vi "ziSetValueDouble.vi"(3 "Error In":errorcluster, 4 "Value":dbl, 5 "Path":string, 6 "Handle In":T1 {"Handle" format="0x%08x"; "Conn" format="0x%08x"}) -> (0 "Error Out":errorcluster, 2 "Handle Out":T1 {"Handle" format="0x%08x"; "Conn" format="0x%08x"})   [LabVIEW 2018, in "Zurich Instruments LabOne.lvlib"]
doc: "This vi sets values to the nodes specified in Path to Value. More than one node can be set if a wildcard is used in Path."
uses:
  Zurich Instruments LabOne.lvlib
  ziTypeHandle.ctl
  ziLV32.dll
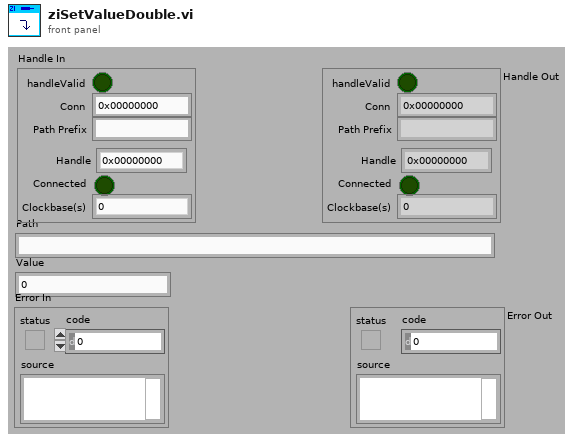
[diagram p1: front panel]
types:
  T1 = typedef "Zurich Instruments LabOne.lvlib/ziTypeHandle.ctl" = cluster{"handleValid":bool, "Conn":u64, "Path Prefix":string, "Handle":u64, "Connected":bool, "Clockbase(s)":dbl}
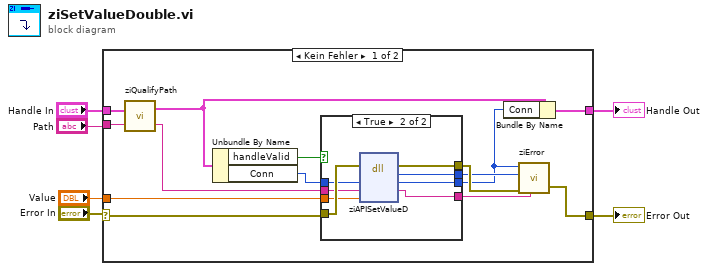
[diagram p0: block diagram]
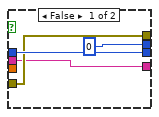
[diagram p2: hidden frame]
diagram:
  n1 = case shown="Kein Fehler" "Error In" {
    selector: "Error In" -> [w8 w34]
    tunnel: "Value" -> [w19 _]
    tunnel: [w18 w34] -> w5
    tunnel: [w14 w33] -> w4
    tunnel: "Handle In" -> [w13 w33]
    tunnel: "Path" -> [w11 _]
    frame No Error {
      n2 = call "ziQualifyPath.vi"("Path In"=w11, "Handle In"=w13) -> ("Path Out"=w10:string, "Handle Out"=w12:T1)
      n3 = Unbundle By Name(w12) -> ("handleValid"=w15:bool, "Conn"=w20:u64)
      n4 = case shown="True" w15 {
        tunnel: w8 -> [w23 w32]
        tunnel: w20 -> [w24 w31]
        tunnel: w10 -> [w21 w30]
        tunnel: w19 -> [_ w29]
        tunnel: [w23 w28] -> w17
        tunnel: [u32 0 ("return type") w27] -> w16
        tunnel: [w24 w26] -> w7
        tunnel: [w21 w25] -> w9
        frame False {
        }
        frame True {
          n5 = dll-call lib="ziLV*.*" fn="ziAPISetValueD"(error in=w32, "Conn"=w31, "Path"=w30, "Value"=w29) -> (error out=w28:errorcluster, "return type"=w27:u32, "Conn"=w26:u64, "Path"=w25:string)  [unwired: 3 in, 1 out]
        }
      }
      n6 = Bundle By Name(cluster=w12, "Conn"=w7) -> (w14:T1)
      n7 = call "ziError.vi"("Conn"=w7, "ziErrorCode"=w16, "Error In"=w17, "Annotation"=w9) -> ("Error Out"=w18:errorcluster)  [unwired: 1 in, 1 out]
    }
    frame Error {
    }
  }
  "Error Out" <- w5
  "Handle Out" <- w4
